vi "SENS_SWE_TIME.vi"(0 "VISA IN":refnum<visa-resource-name>, 1 "Sweep Time(sec)":dbl, 5 "error in":errorcluster, 7 "Channel":i32) -> (14 "VISA Out":refnum<visa-resource-name>, 19 "error out":errorcluster)   [LabVIEW 2018, in "PNA-X.lvlib"]
doc: "SENSe<cnum>:SWEep:TIME <num> \n(Read-Write) Sets the time the analyzer takes to complete one sweep. If sweep time accuracy is critical, use \nONLY the values that are attained using the up and down arrows next to the sweep time entry box. See Sweep \nTime. \nParameters \n<cnum> Any existing channel number. If unspecified, value is set to 1 \n<num> Sweep time in seconds. Choose a number between 0 and 86,400 (24hrs), \nTo select the fastest sweep speed, either send MIN as an argument to this command, or \nsend SENS:SWE:TIME:AUTO 1 \nSee Note \nExamples SENS:SWE:TIME 1ms \nsense2:sweep:time .001 \nQuery Syntax SENSe<cnum>:SWEep:TIME? \nReturn Type Numeric \nDefault NA"
uses:
  PNA-X.lvlib
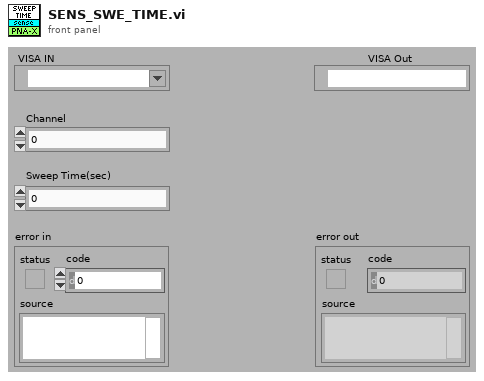
[diagram p1: front panel]
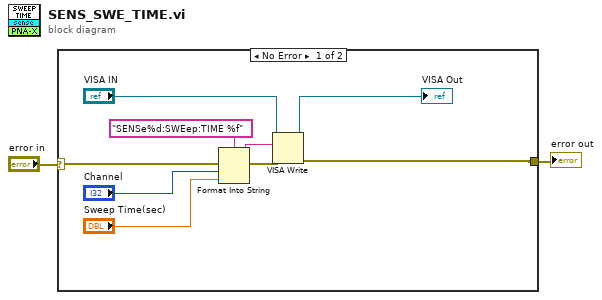
[diagram p0: block diagram]
diagram:
  n1 = case shown="No Error" "error in" {
    selector: "error in" -> [w11 w12]
    tunnel: [w6 w12] -> w1
    frame No Error {
      n2 = Format Into String(format string="SENSe%d:SWEep:TIME %f" ("Cmdline"), error in=w11, "Channel", "Sweep Time(sec)") -> (resulting string=w9:string, error out=w10:errorcluster)  [unwired: 1 in]
      n3 = VISA Write(VISA resource name="VISA IN", write buffer=w9, error in (no error)=w10) -> (VISA resource name out=→"VISA Out":refnum<visa-resource-name>, error out=w6:errorcluster)  [unwired: 1 out]
    }
    frame Error {
    }
  }
  "error out" <- w1
